vi "ApplyScalePost.vi"(8 "error in (no error)":errorcluster, 10 "Y Array":sgl[](array[numeric]), 11 "RTD in":refnum<class "RTD.lvclass">) -> (0 "error out":errorcluster, 2 "Y Array":sgl[](array[numeric]), 3 "RTD out":refnum<class "RTD.lvclass">)   [LabVIEW 2018, in "Measurement Channels.lvlib" / "RTD.lvclass"]
uses:
  RTD.lvclass
  C:/Users/Jeff Tipps/Documents/DAQMan/source/Classes/Measurements/Class Channel/Channel.lvclass
  Class Channel/Read Scale.vi
  Class Channel/Read Offset.vi
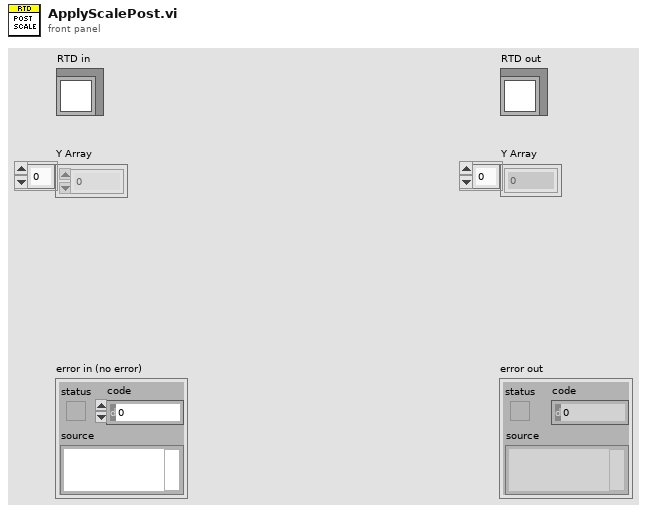
[diagram p1: front panel]
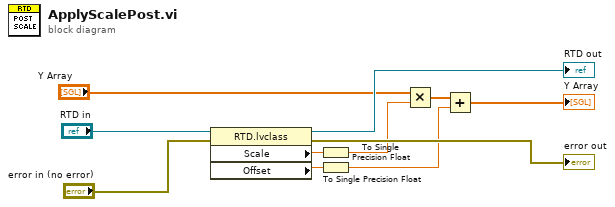
[diagram p0: block diagram]
diagram:
  n1 = property class="RTD.lvclass"(reference="RTD in", error in="error in (no error)") -> (reference out=→"RTD out":refnum<class "RTD.lvclass">, error out=→"error out":errorcluster, "Scale"=w7:dbl, "Offset"=w6:dbl)
  n2 = To Single Precision Float(number=w7) -> (single precision float=w4:sgl)
  n3 = To Single Precision Float(number=w6) -> (single precision float=w2:sgl)
  n4 = Multiply(x="Y Array", y=w4) -> (x*y=w3:sgl[])
  n5 = Add(x=w3, y=w2) -> (x+y=→"Y Array":sgl[])
